vi "Close.vi"(8 "error in":errorcluster, 11 "SpreadsheetDoc":refnum<k24>) -> (0 "error out":errorcluster)   [LabVIEW 2019, in "Open Xml.lvlib"]
uses:
  Open Xml.lvlib
  D:/git/Open-Xml-LabVIEW/Source/DocumentFormat.OpenXml.dll
  DocumentFormat.OpenXml.dll
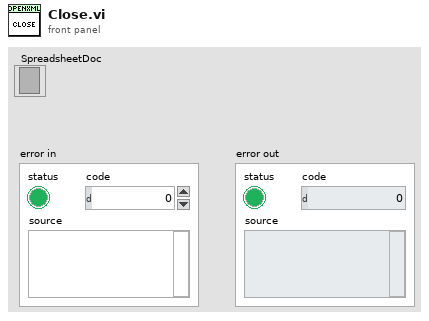
[diagram p1: front panel]
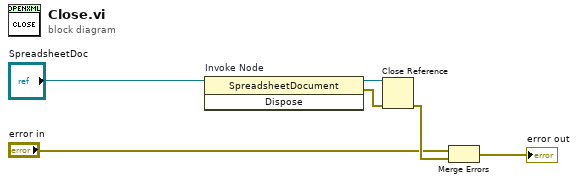
[diagram p0: block diagram]
diagram:
  n1 = invoke on="Invoke Node" class="SpreadsheetDocument" method="Dispose"(reference="SpreadsheetDoc") -> (reference out=w4:refnum<k24>, error out=w3:errorcluster)  [unwired: 2 in, 1 out]
  n2 = Close Reference(reference=w4, error in (no error)=w3) -> (error out=w6:errorcluster)
  n3 = Merge Errors("error in", w6) -> (→"error out":errorcluster)
